vi "sub_prepare_HexPlot_command.vi"(10 "Dynamic data":T1, 11 "Input parameters":T2={"Measurement type"=enum."Debug", "Sensor type"=enum."HPK_8in_256", "Identifier"="test.txt", "Open after execution?"=FALSE, "Plot after execution?"=FALSE, "Display channel"=0, "Voltage Delay (s)"=0.5, "Switch Delay (s)"=0.01, "VISA resource name source"="", "VISA resource name DMM"="", "VISA resource name LCR"="", "Compliance  Level (A)"=10.0, "Voltage Limit (V)"=1000.0, "Data storage location"="", "Scan voltages"="", "Use source as DMM?"=FALSE, "LCR signal frequenzy (Hz)"=10.0, "DMM device"=enum."Keithley2001", "Sampling number"=1, "Use env. sensors on"=enum."Sensirion sht1x/7x", "Switchboard Handle"=0, "Use Switchboard"=FALSE, "LCR signal voltage (V)"=10000.0, "Repeat"=1, "Scan voltages IV"="", "Scan voltages CV"="", "Hex pad numbers?"=FALSE, "Set measurement type"=enum."Debug", "Custom pad scan"="", "IV voltage Delay (s)"=0.5, "CV voltage Delay (s)"=0.5, "Needle measurement?"=FALSE, "Comments"="test.txt", "LCR signal frequenzy (kHz)"=10.0, "Compliance  Level (uA)"=10.0, "Open Correction Array"=array2304x3[6912 elements], "Current set voltage"=0.0, "Last set voltage"=0.0, "Current channel"=0, "Last OpenCorrection index"=-1, "Total curr/vltg every x steps"=10, "Current channel iteration"=0, "No CV corrections"=FALSE, "Mapfile"="", "Corrfile"="", "IV voltage file"=path "", "CV voltage file"=path "", "IV Switch Delay (s)"=0.01, "CV Switch Delay (s)"=0.01, "Invert polarity"=FALSE, "Set debug dirs"=FALSE, "Is n on p"=FALSE} {"CV Switch Delay (s)" format="%#_13g"; "IV Switch Delay (s)" format="%#_13g"; "Last set voltage" format="%#_13g"; "Current set voltage" format="%#_13g"; "CV voltage Delay (s)" format="%#_13g"; "IV voltage Delay (s)" format="%#_13g"; "Voltage Limit (V)" format="%#_13g"; "Voltage Delay (s)" format="%#_13g"; "Switch Delay (s)" format="%#_13g"}) -> (2 "Dynamic data out":T1)   [LabVIEW 2016]
doc: "Set HexPlot command for data display."
uses:
  input_params.ctl
  data_dynamic.ctl
panel:
  out "HexPlot matrix command":string
  out "HexPlot command":string
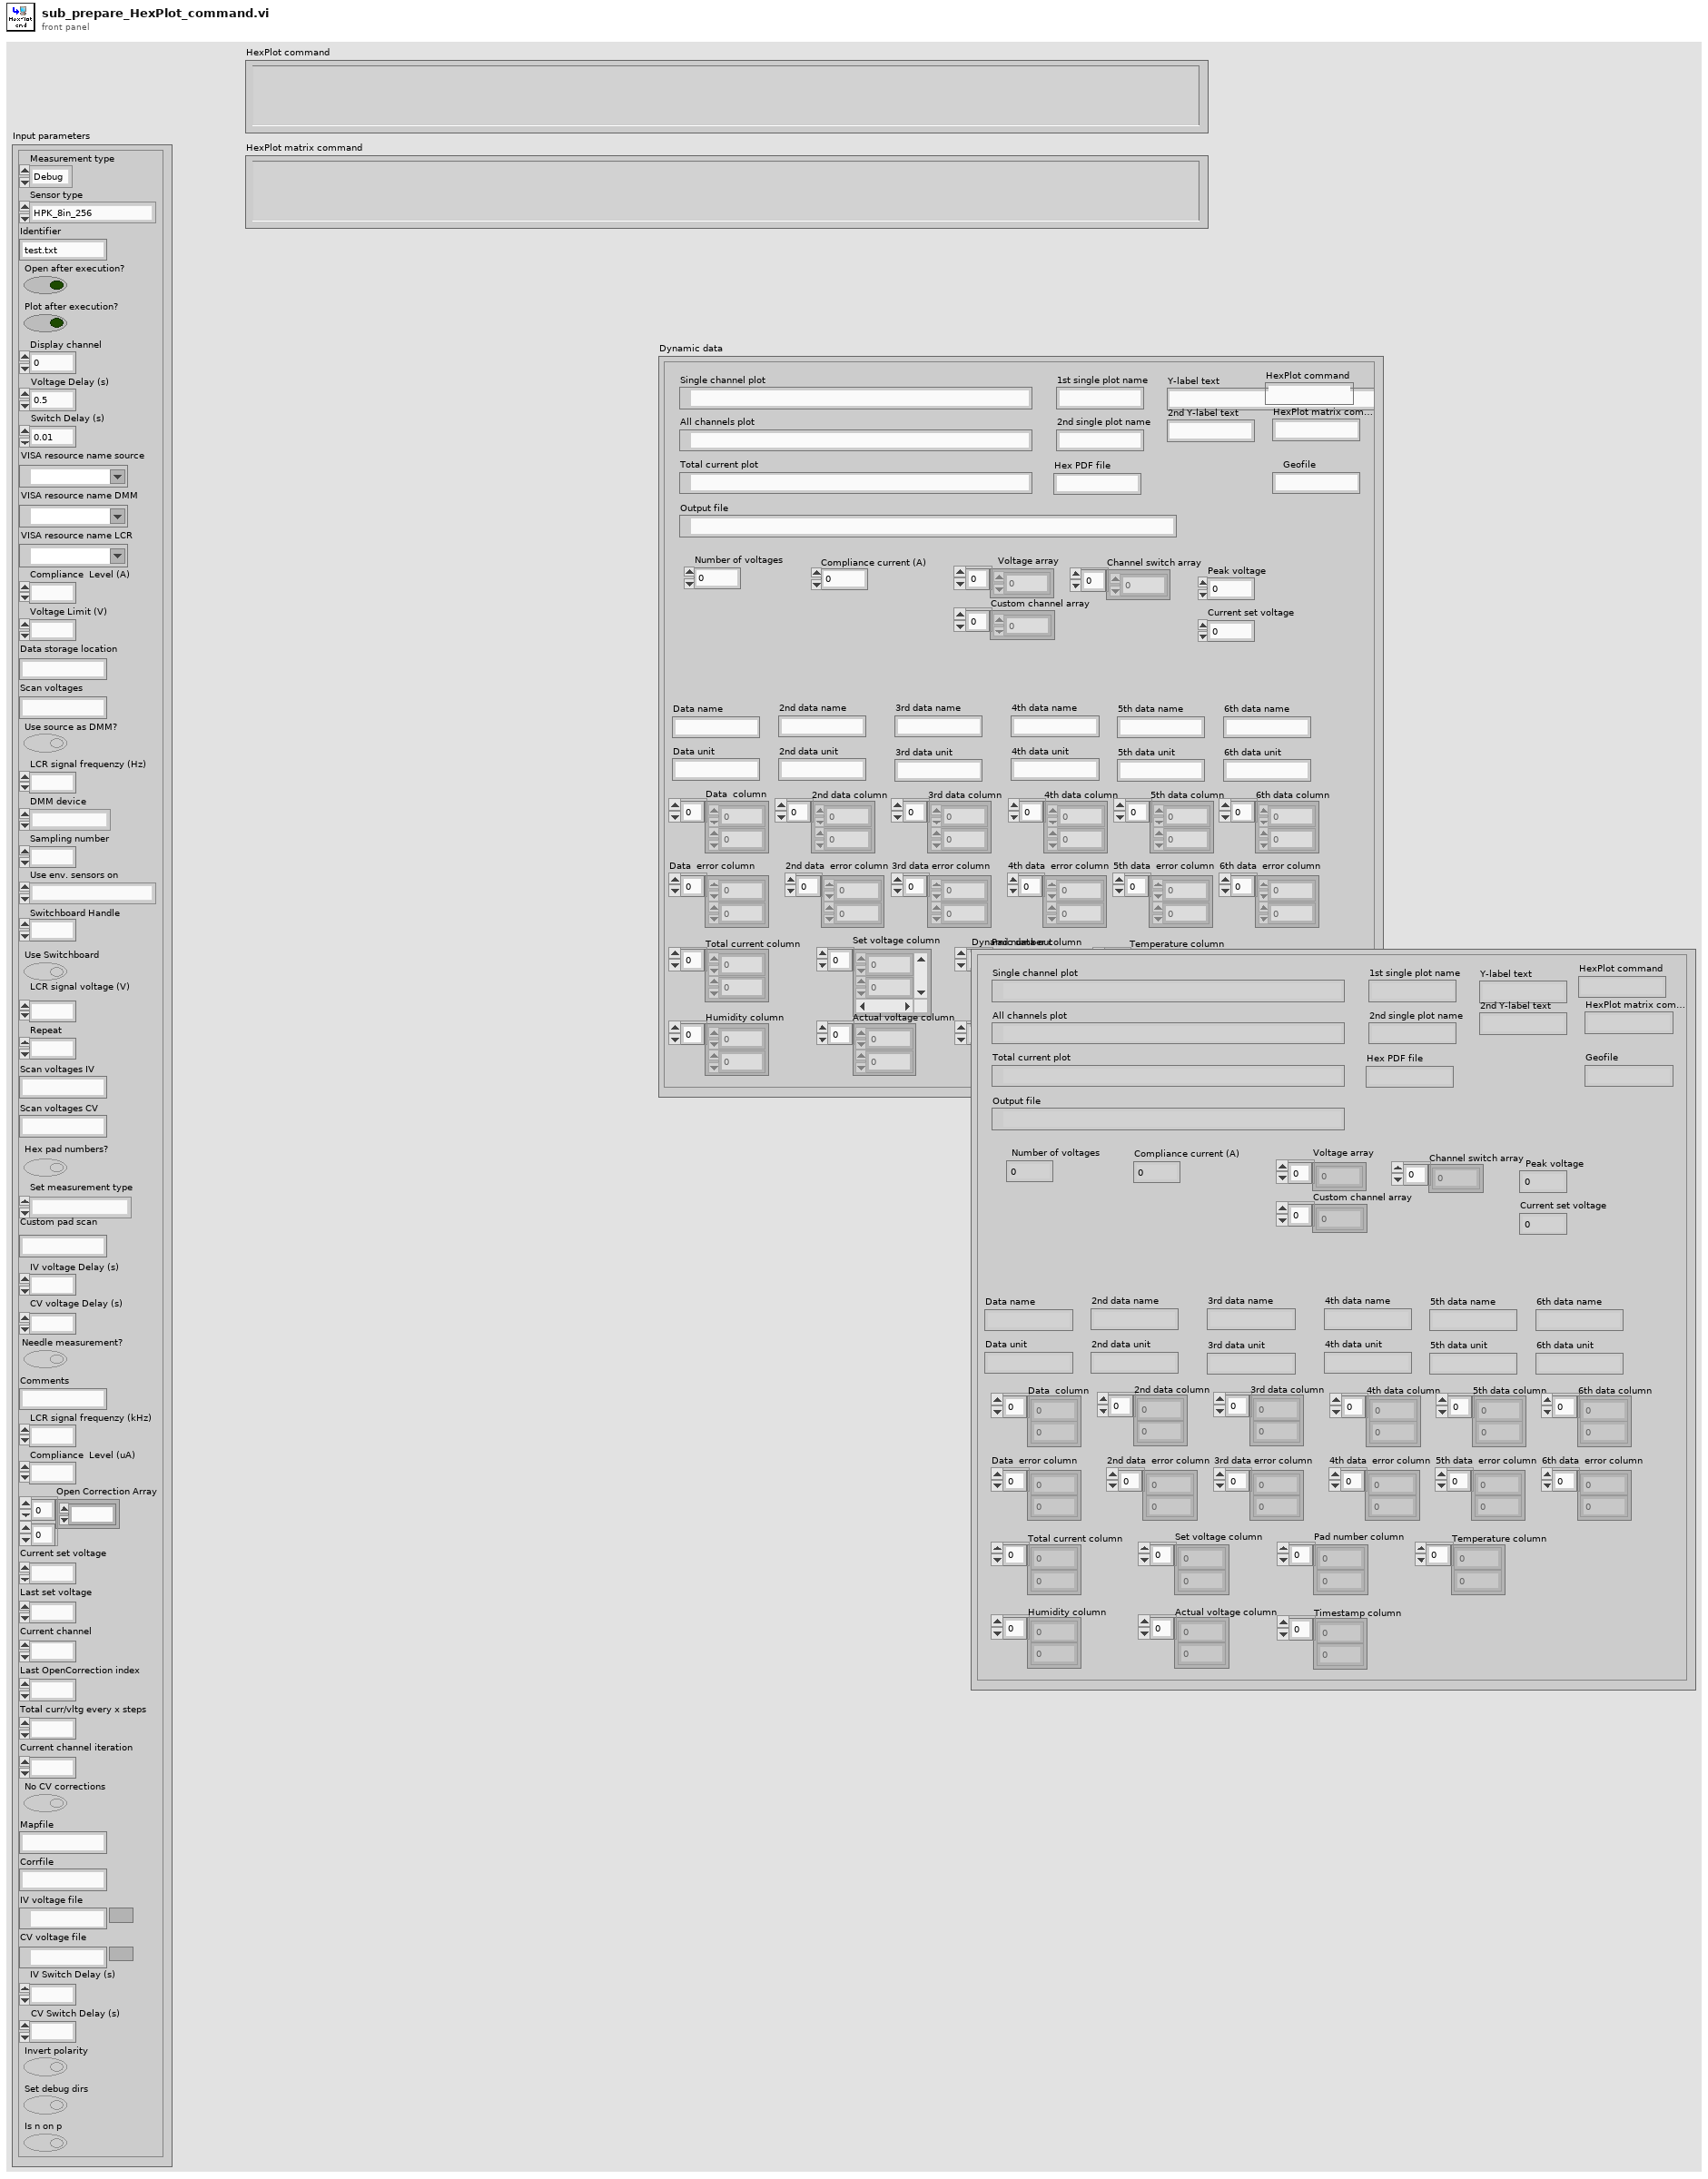
[diagram p1: front panel]
types:
  T1 = typedef "data_dynamic.ctl" = cluster{"Output file":path, "Y-label text":string, "Current set voltage":dbl, "Set voltage column":dbl[], "Pad number column":dbl[], "Data  column":dbl[], "Number of voltages":i32, "Compliance current (A)":dbl, "Geofile":string, "Peak voltage":dbl, "Hex PDF file":string, "Voltage array":dbl[], "Total current column":dbl[], "Timestamp column":dbl[], "Data name":string, "Data unit":string, "2nd data column":dbl[], "2nd data name":string, "2nd data unit":string, "3rd data column":dbl[], "4th data column":dbl[], "3rd data name":string, "3rd data unit":string, "4th data name":string, "4th data unit":string, "Actual voltage column":dbl[], "2nd Y-label text":string, "Single channel plot":path, "Temperature column":dbl[], "Humidity column":dbl[], "Channel switch array":i32[], "1st single plot name":string, "2nd single plot name":string, "All channels plot":path, "HexPlot command":string, "Custom channel array":i32[], "Data  error column":dbl[], "2nd data  error column":dbl[], "3rd data error column":dbl[], "4th data  error column":dbl[], "Total current plot":path, "5th data column":dbl[], "5th data  error column":dbl[], "6th data column":dbl[], "6th data  error column":dbl[], "5th data name":string, "5th data unit":string, "6th data name":string, "6th data unit":string, "HexPlot matrix command":string}
  T2 = typedef "input_params.ctl" = cluster{"Measurement type":enum16{"IV", "CV", "Debug", "Test_contact"}, "Sensor type":enum16{"HPK_6in_135", "HPK_8in_256", "IFX_8in_256", "Diode", "HPK_6in_256", "Full matrix"}, "Identifier":string, "Open after execution?":bool, "Plot after execution?":bool, "Display channel":i32, "Voltage Delay (s)":dbl, "Switch Delay (s)":dbl, "VISA resource name source":refnum<visa-resource-name>, "VISA resource name DMM":refnum<visa-resource-name>, "VISA resource name LCR":refnum<visa-resource-name>, "Compliance  Level (A)":dbl, "Voltage Limit (V)":dbl, "Data storage location":string, "Scan voltages":string, "Use source as DMM?":bool, "LCR signal frequenzy (Hz)":dbl, "DMM device":enum16{"Keithley2001", "Keithley2450", "Keithley2410", "Keithley6487"}, "Sampling number":i32, "Use env. sensors on":enum16{"Sensirion sht1x/7x", "Switch Matrix", "Probecard"}, "Switchboard Handle":u32, "Use Switchboard":bool, "LCR signal voltage (V)":dbl, "Repeat":i32, "Scan voltages IV":string, "Scan voltages CV":string, "Hex pad numbers?":bool, "Set measurement type":enum16{"IV", "CV", "Debug", "Test_contact", "IV+CV"}, "Custom pad scan":string, "IV voltage Delay (s)":dbl, "CV voltage Delay (s)":dbl, "Needle measurement?":bool, "Comments":string, "LCR signal frequenzy (kHz)":dbl, "Compliance  Level (uA)":dbl, "Open Correction Array":dbl[][], "Current set voltage":dbl, "Last set voltage":dbl, "Current channel":i32, "Last OpenCorrection index":i32, "Total curr/vltg every x steps":i32, "Current channel iteration":i32, "No CV corrections":bool, "Mapfile":string, "Corrfile":string, "IV voltage file":path, "CV voltage file":path, "IV Switch Delay (s)":dbl, "CV Switch Delay (s)":dbl, "Invert polarity":bool, "Set debug dirs":bool, "Is n on p":bool}
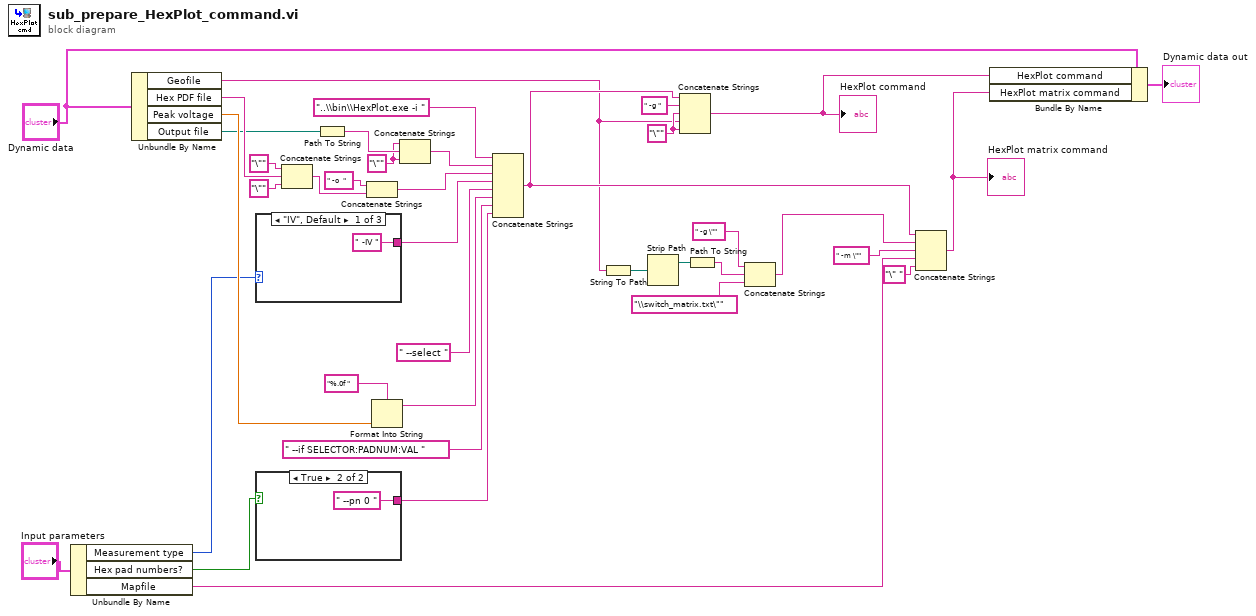
[diagram p0: block diagram]
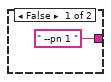
[diagram p2: hidden frame]
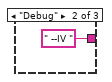
[diagram p3: hidden frame]
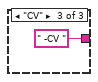
[diagram p4: hidden frame]
diagram:
  w13 = "\"" ("string")
  w12 = "\"" ("string")
  n1 = Unbundle By Name("Input parameters") -> ("Measurement type"=w24:enum16{"IV", "CV", "Debug", "Test_contact"}, "Hex pad numbers?"=w21:bool, "Mapfile"=w14:string)
  n2 = Unbundle By Name("Dynamic data") -> ("Geofile"=w8:string, "Hex PDF file"=w25:string, "Peak voltage"=w35:dbl, "Output file"=w22:path)
  n3 = case shown="\"IV\", Default" w24 {
    tunnel: [" -IV " ("string") " --IV " ("string") " -CV " ("string")] -> w37
    frame "IV", Default {
    }
    frame "Debug" {
    }
    frame "CV" {
    }
  }
  n4 = case shown="True" w21 {
    tunnel: [" --pn 1 " ("string") " --pn 0 " ("string")] -> w20
    frame False {
    }
    frame True {
    }
  }
  n5 = Concatenate Strings("\"" ("string"), w25, "\"" ("string")) -> (w26:string)
  n6 = Path To String(path=w22) -> (string=w23:string)
  n7 = Concatenate Strings(" -o  " ("string"), w26) -> (w30:string)
  n8 = Format Into String(format string="%.0f ", w35) -> (resulting string=w33:string)  [unwired: 2 in, 1 out]
  n9 = Concatenate Strings(w13, w23, w13) -> (w31:string)
  n10 = Concatenate Strings("..\\bin\\HexPlot.exe -i " ("string"), w31, w30, w37, " --select " ("string"), w33, " --if SELECTOR:PADNUM:VAL " ("string"), w20) -> (w9:string)
  n11 = String To Path(string=w8) -> (path=w7:path)
  n12 = Strip Path(path=w7) -> (stripped path=w6:path)  [unwired: 1 out]
  n13 = Concatenate Strings(w9, " -g " ("string"), w12, w8, w12) -> (w10:string)
  "HexPlot command" <- w10
  n14 = Path To String(path=w6) -> (string=w5:string)
  n15 = Concatenate Strings(" -g \"" ("string"), w5, "\\switch_matrix.txt\"" ("string")) -> (w3:string)
  n16 = Concatenate Strings(w9, w3, " -m \"" ("string"), w14, "\" " ("string")) -> (w1:string)
  "HexPlot matrix command" <- w1
  n17 = Bundle By Name(cluster="Dynamic data", "HexPlot command"=w10, "HexPlot matrix command"=w1) -> (→"Dynamic data out":T1)
